vi "Read pdoBufferSize.vi"(8 "error in (no error)":errorcluster, 11 "OrionBMS in":refnum<class "OrionBMSClass.lvclass">) -> (0 "error out":errorcluster, 2 "pdoBufferSize":u16, 3 "OrionBMS out":refnum<class "OrionBMSClass.lvclass">)   [LabVIEW 2018, in "OrionBMSClass.lvclass"]
uses:
  OrionBMSClass.lvclass
  OrionBMSClass.lvclass/OrionBMSClass.ctl
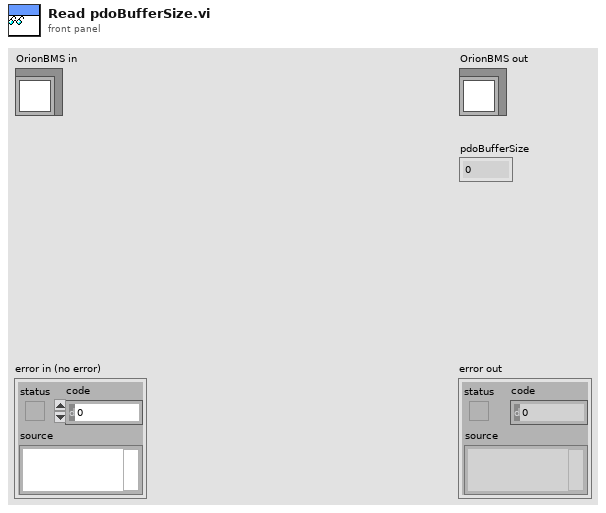
[diagram p1: front panel]
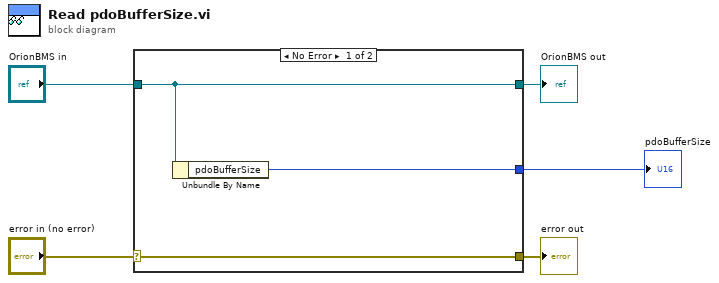
[diagram p0: block diagram]
diagram:
  n1 = case shown="No Error" "error in (no error)" {
    selector: "error in (no error)" -> [w8 w9]
    tunnel: [w8 w9] -> w4
    tunnel: [w7 w10] -> w2
    tunnel: "OrionBMS in" -> [w7 w10]
    tunnel: [w6 _] -> w1
    frame No Error {
      n2 = Unbundle By Name(w7) -> ("pdoBufferSize"=w6:u16)
    }
    frame Error {
    }
  }
  "error out" <- w4
  "OrionBMS out" <- w2
  "pdoBufferSize" <- w1
